vi "Wait_Return_IHM.vi"(8 "error in (no error)":errorcluster caption="entrée d'erreur (pas d'erreur)", 11 "Class Popup (Default) en entrée":refnum<class "Class Popup (Main).lvclass">) -> (0 "error out":errorcluster caption="sortie d'erreur", 3 "Class Popup (Default) en sortie":refnum<class "Class Popup (Main).lvclass">)   [LabVIEW 2020, in "Library Instrument & Equipement.lvlib" / "Library Popup.lvlib" / "Class Popup (Main).lvclass"]
uses:
  Class Popup (Main).lvclass
  Class Popup (Main).lvclass/Class Popup (Main).ctl
  Commun VI/Library Commun.lvlib
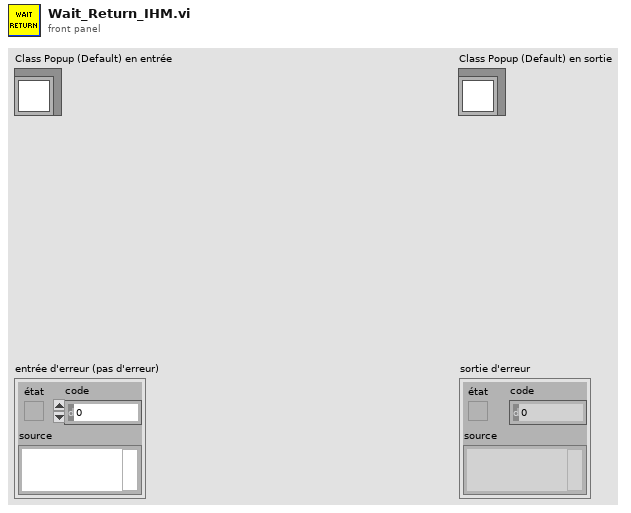
[diagram p1: front panel]
types:
  T1 = enum16{"Get Variable", "Get All Variables", "Set Variable", "Delete Variable", "Delete All Variable"}
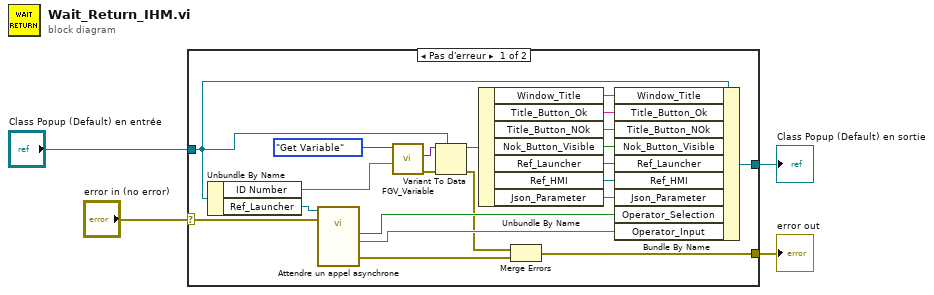
[diagram p0: block diagram]
diagram:
  n1 = case shown="Pas d'erreur" "error in (no error)" {
    selector: "error in (no error)" -> [w24 w27]
    tunnel: [w22 w27] -> w3
    tunnel: [w21 w26] -> w1
    tunnel: "Class Popup (Default) en entrée" -> [w14 w26]
    frame No Error {
      n2 = Unbundle By Name(w14) -> ("ID Number"=w18:string, "Ref_Launcher"=w25:refnum<vi>)
      n3 = call-by-ref "Attendre un appel asynchrone"(reference=w25, error in=w24) -> ("error out"=w23:errorcluster, "Input"=w19:string, "Operator_Selection"=w20:bool)  [unwired: 9 in, 2 out]
      n4 = call "FGV_Variable.vi"("Variable"=w18, "Function"=T1."Get Variable") -> ("error out"=w16:errorcluster, "Data Out"=w13:variant)  [unwired: 7 in, 1 out]
      n5 = Variant To Data(error in=w16, type=w14, Variant=w13) -> (data=w12:refnum<class "Class Popup (Main).lvclass">, error out=w15:errorcluster)
      n6 = Unbundle By Name(w12) -> ("Window_Title"=w11:string, "Title_Button_Ok"=w10:string, "Title_Button_NOk"=w9:string, "Nok_Button_Visible"=w8:bool, "Ref_Launcher"=w7:refnum<vi>, "Ref_HMI"=w6:refnum<vi>, "Json_Parameter"=w5:string)
      n7 = Merge Errors(w15, w23) -> (w22:errorcluster)
      n8 = Bundle By Name(cluster=w14, "Window_Title"=w11, "Title_Button_Ok"=w10, "Title_Button_NOk"=w9, "Nok_Button_Visible"=w8, "Ref_Launcher"=w7, "Ref_HMI"=w6, "Json_Parameter"=w5, "Operator_Selection"=w20, "Operator_Input"=w19) -> (w21:refnum<class "Class Popup (Main).lvclass">)
    }
    frame Error {
    }
  }
  "error out" <- w3
  "Class Popup (Default) en sortie" <- w1
